vi "Sum roman numerial numeric array.vi"(8 "error in (no error)":errorcluster, 11 "Roman numeral array":i32[](array[numeric])) -> (0 "error out":errorcluster, 3 "Summed array":i32)   [LabVIEW 2023]
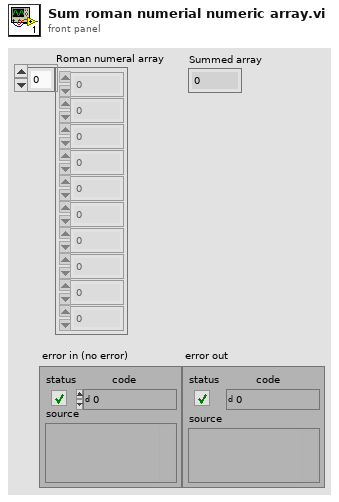
[diagram p1: front panel]
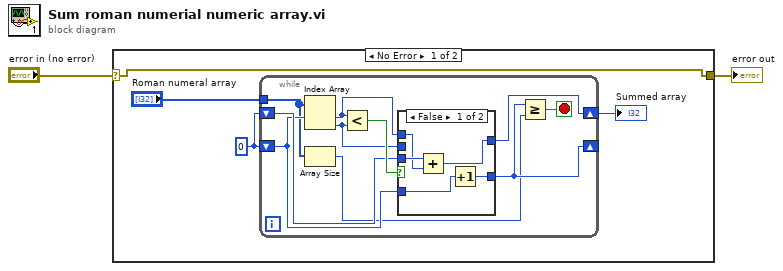
[diagram p0: block diagram]
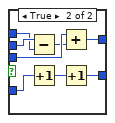
[diagram p2: hidden frame]
diagram:
  n1 = case shown="No Error" "error in (no error)" {
    selector: "error in (no error)" -> [w3 w30]
    tunnel: [w3 w30] -> w1
    frame No Error {
      w6 = 0
      n2 = while {
        tunnel: "Roman numeral array" -> [w8]
        shift-right: [w10] -> _
        shift-left: w6 -> [w11]
        shift-right: [w13] -> w4
        shift-left: w6 -> [w12]
        stop <- w9 stop-if-true
        n3 = Index Array(array=w8, index #1=w11) -> (element #1=w15:i32, element #2=w14:i32)  [unwired: 1 in]
        n4 = Array Size(array=w8) -> (size(s)=w7:i32)
        n5 = Less?(x=w15, y=w14) -> (x < y?=w16:bool)
        n6 = case shown="False" w16 {
          tunnel: w15 -> [w19 w28]
          tunnel: w14 -> [_ w29]
          tunnel: [w20 w26] -> w13
          tunnel: w12 -> [w21 w27]
          tunnel: w11 -> [w18 w24]
          tunnel: [w17 w22] -> w10
          frame False {
            n7 = Add(x=w21, y=w19) -> (x+y=w20:i32)
            n8 = Increment(x=w18) -> (x+1=w17:i32)
          }
          frame True {
            n9 = Subtract(x=w29, y=w28) -> (x-y=w25:i32)
            n10 = Increment(x=w24) -> (x+1=w23:i32)
            n11 = Add(x=w27, y=w25) -> (x+y=w26:i32)
            n12 = Increment(x=w23) -> (x+1=w22:i32)
          }
        }
        n13 = Greater Or Equal?(x=w10, y=w7) -> (x >= y?=w9:bool)
      }
      "Summed array" <- w4
    }
    frame Error {
    }
  }
  "error out" <- w1
